vi "UI Main.vi"() -> ()   [LabVIEW 2013]
uses:
  controls/UI Data.ctl
  Globals/Global - All UI Loop Stop.vi
  support/Message Queue/Message Queue.lvlib
  support/User Event - Stop/User Event - Stop.lvlib
panel:
  out "Error Infomation":string caption="错误信息"
  in  "Connect to Controller":bool caption="连接控制器"
  out "Controller Operating Status":u16(ring)=1 caption="控制器运行状态" items=["采集与记录", "安全状态"]
  out "Connected?":bool caption="已连接？"
  in  "Controller Address":string="169.254.4.42" caption="控制器地址"
  in  "Settings Tab":enum32{"采集与记录", "System Monitoring"}(tab) caption="设置选项卡"
  in  "Manually Trigger Data Logging":bool caption="人为触发数据采集"
  out "Live Data":waveform(dbl)[](graph) caption="实时数据"
  in  "Acquire Live Data":bool caption="获取实时数据"
  out "Latest Data Logging File":path=path "最新数据记录文件" caption="最新数据记录文件"
  out "Number of Data Files":u32 caption="数据文件数："
  out "Actual Loop Period (ticks)":u32 caption="实际循环周期（时钟滴答）："
  out "Largest Contiguous Memory (bytes)":dbl(graph) caption="最大连续内存（字节）"
  out "System Time":timestamp caption="系统时间" format="%<%Y/%m/%d %H:%M:%S>T"
  out "Resource Utilization (%)":T1(graph) caption="资源利用率(%)"
  in  "Exit":bool caption="退出"
  # "CompactRIO上的LabVIEW FPGA波形采集与记录"
  # "连接设置"
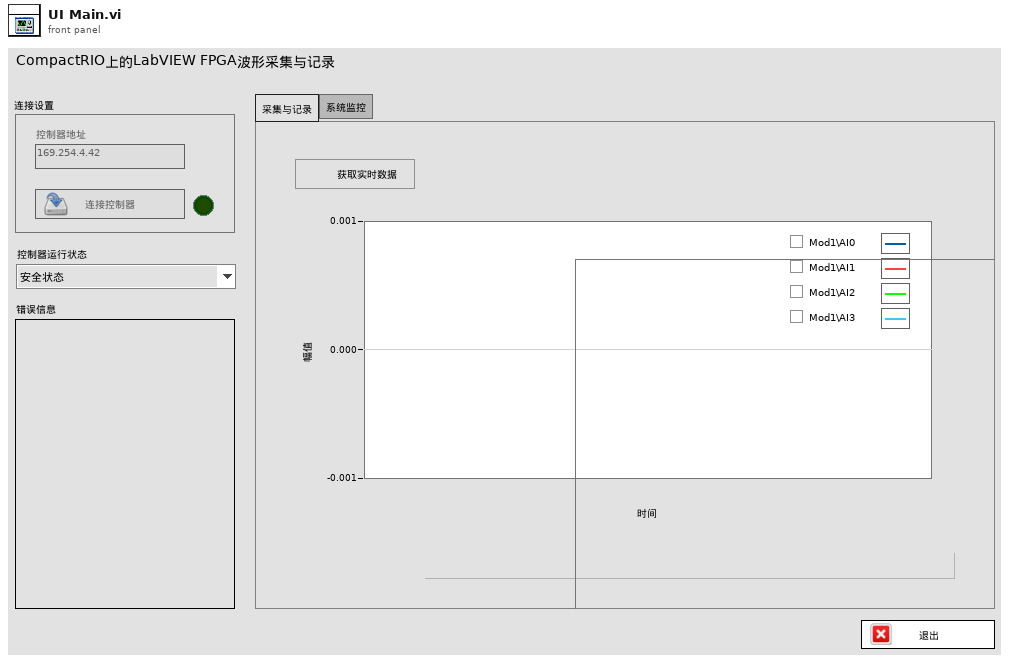
[diagram p1: front panel]
types:
  T1 = cluster{"CPU Usage":dbl, "Buffer Backlog":dbl, "Driver Space":dbl}
  T2 = typedef "UI Data.ctl" = cluster{"Connect to Controller Ref":refnum<vi>, "Connected? Ref":refnum<vi>, "Manually Trigger Data Logging Ref":refnum<vi>, "Acquire Live Data Ref":refnum<vi>, "Stop Live Data Ref":refnum<vi>, "Exit":refnum<vi>, "Controller Address Ref":refnum<vi>, "Error Infomation Ref":refnum<vi>, "Latest Data Logging File Ref":refnum<vi>, "Current Logging State Ref":refnum<vi>, "Actual Loop Period (ticks) Ref":refnum<vi>, "Number of Data Files Ref":refnum<vi>, "System Time Ref":refnum<vi>, "Contiguous Memory Ref":refnum<vi>, "Resource Utilization (%) Ref":refnum<vi>, "Live Data Ref":refnum<vi>, "Setting Tab Ref ":refnum<vi>}
  T3 = typedef "Message Queue.lvlib/All Host Message Queues.ctl" = cluster{"UI":refnum<queue>}
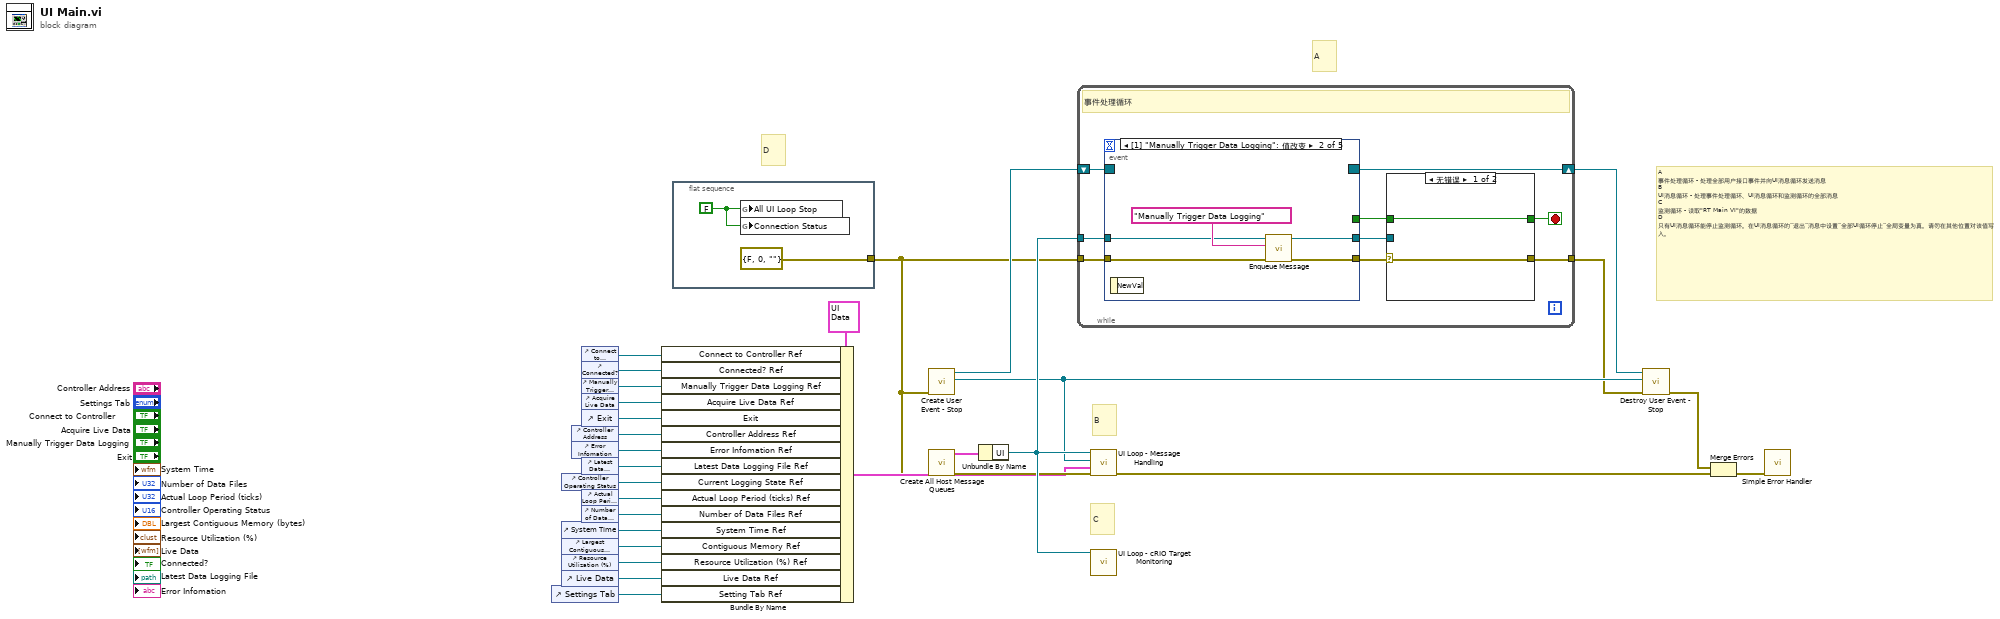
[diagram p0: block diagram]
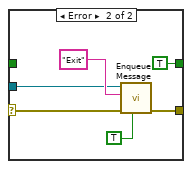
[diagram p2: hidden frame]
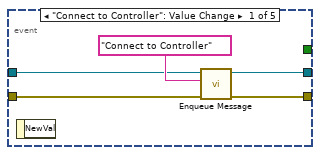
[diagram p3: hidden frame]
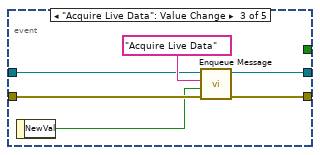
[diagram p4: hidden frame]
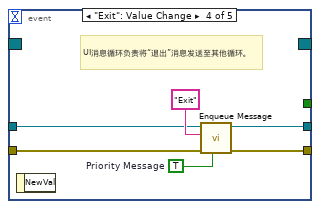
[diagram p5: hidden frame]
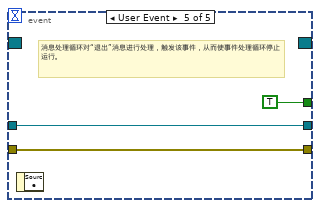
[diagram p6: hidden frame]
diagram:
  # "C"
  # "A"
  # "B"
  # "D"
  # "A\n事件处理循环 - 处理全部用户接口事件并向UI消息循环发送消息\nB\nUI消息循环 - 处理事件处理循环、UI消息循环和监测循环的全部消息\nC\n监测循环 - 读取\"RT Main VI\"的数据\nD\n只有UI消息循环能停止监测循环。在UI消息循环的“退出”消息中设置“全部UI循环停止”全局变量为真。请勿在其他位置对该值写入。"
  n1 = control-ref of="Settings Tab"() -> (w1:refnum<vi>)
  n2 = control-ref of="Controller Operating Status"() -> (w8:refnum<vi>)
  n3 = control-ref of="System Time"() -> (w5:refnum<vi>)
  n4 = control-ref of="Largest Contiguous Memory (bytes)"() -> (w4:refnum<vi>)
  n5 = control-ref of="Resource Utilization (%)"() -> (w3:refnum<vi>)
  n6 = control-ref of="Live Data"() -> (w2:refnum<vi>)
  n7 = control-ref of="Controller Address"() -> (w18:refnum<vi>)
  n8 = control-ref of="Error Infomation"() -> (w9:refnum<vi>)
  n9 = control-ref of="Connect to Controller"() -> (w23:refnum<vi>)
  n10 = control-ref of="Connected?"() -> (w22:refnum<vi>)
  n11 = control-ref of="Manually Trigger Data Logging"() -> (w21:refnum<vi>)
  n12 = control-ref of="Acquire Live Data"() -> (w20:refnum<vi>)
  n13 = control-ref of="Exit"() -> (w19:refnum<vi>)
  n14 = control-ref of="Latest Data Logging File"() -> (w17:refnum<vi>)
  n15 = control-ref of="Actual Loop Period (ticks)"() -> (w7:refnum<vi>)
  n16 = control-ref of="Number of Data Files"() -> (w6:refnum<vi>)
  n17 = Bundle By Name(cluster=T2 {"Connect to Controller Ref"=refnum, "Connected? Ref"=refnum, "Manually Trigger Data Logging Ref"=refnum, "Acquire Live Data Ref"=refnum, "Stop Live Data Ref"=refnum, "Exit"=refnum, "Controller Address Ref"=refnum, "Error Infomation Ref"=refnum, "Latest Data Logging File Ref"=refnum, "Current Logging State Ref"=refnum, "Actual Loop Period (ticks) Ref"=refnum, "Number of Data Files Ref"=refnum, "System Time Ref"=refnum, "Contiguous Memory Ref"=refnum, "Resource Utilization (%) Ref"=refnum, "Live Data Ref"=refnum, "Setting Tab Ref "=refnum} ("Measurement UI Controls"), "Connect to Controller Ref"=w23, "Connected? Ref"=w22, "Manually Trigger Data Logging Ref"=w21, "Acquire Live Data Ref"=w20, "Exit"=w19, "Controller Address Ref"=w18, "Error Infomation Ref"=w9, "Latest Data Logging File Ref"=w17, "Current Logging State Ref"=w8, "Actual Loop Period (ticks) Ref"=w7, "Number of Data Files Ref"=w6, "System Time Ref"=w5, "Contiguous Memory Ref"=w4, "Resource Utilization (%) Ref"=w3, "Live Data Ref"=w2, "Setting Tab Ref"=w1) -> (w12:T2)
  n18 = flat-sequence {
    tunnel: [errorcluster {"status"=FALSE, "code"=0, "source"=""} ("error in (no error)")] -> w11
    frame #0 {
      w30 = FALSE
      n19 = global write "Global - All UI Loop Stop.vi" "All UI Loop Stop"(w30) -> ()
      n20 = global write "Global - All UI Loop Stop.vi" "Connection Status"(w30) -> ()
    }
  }
  n21 = call "Create User Event - Stop.vi"("error in (no error)"=w11) -> ("User Event - Stop"=w15:refnum<user-event>, "Stop Event Registration Refnum"=w29:refnum<event-registration>)  [unwired: 8 in, 1 out]
  n22 = call "Create All Host Message Queues.vi"("error in (no error)"=w11) -> ("error out"=w26:errorcluster, "Message Queues out"=w28:T3)  [unwired: 9 in]
  n23 = Unbundle By Name(w28) -> ("UI"=w27:refnum<queue>)
  n24 = while {
    tunnel: w27 -> [w36]
    shift-right: [w35] -> w13
    shift-left: w29 -> [w37]
    tunnel: w11 -> [w34]
    tunnel: [w32] -> w10
    stop <- w39 stop-if-true
    # "事件处理循环"
    n25 = event shown="[1] \"Manually Trigger Data Logging\": 值改变" {
      selector: w37 -> [_ _ _ _ _]
      dyn-events: [_ _ _ _ _] -> w35
      timeout: _ -> [_ _ _ _ _]
      tunnel: [_ _ _ _ TRUE ("Discard?")] -> w40
      tunnel: w36 -> [w51 w56 w62 w67 w71]
      tunnel: [w53 w58 w64 w70 w72] -> w38
      tunnel: w34 -> [w50 w55 w61 w66 w72]
      tunnel: [w49 w54 w60 w65 w71] -> w33
      event "Connect to Controller": Value Change {
        n26 = event-data() -> ()  [unwired: 1 in, 1 out]
        n27 = call "Enqueue Message.vi"("error in (no error)"=w50, "Message"="Connect to Controller", "Message Queue"=w51) -> ("error out"=w53:errorcluster, "dup Message Queue"=w49:refnum<queue>)  [unwired: 7 in]
      }
      event "Manually Trigger Data Logging": Value Change {
        n28 = event-data() -> ()  [unwired: 1 in, 1 out]
        n29 = call "Enqueue Message.vi"("error in (no error)"=w55, "Message"="Manually Trigger Data Logging", "Message Queue"=w56) -> ("error out"=w58:errorcluster, "dup Message Queue"=w54:refnum<queue>)  [unwired: 7 in]
      }
      event "Acquire Live Data": Value Change {
        n30 = event-data() -> ("NewVal"=w59:bool)  [unwired: 1 in]
        n31 = call "Enqueue Message.vi"("error in (no error)"=w61, "Message Data"=w59, "Message"="Acquire Live Data", "Message Queue"=w62) -> ("error out"=w64:errorcluster, "dup Message Queue"=w60:refnum<queue>)  [unwired: 6 in]
      }
      event "Exit": Value Change {
        w68 = TRUE  # Priority Message
        # "UI消息循环负责将“退出”消息发送至其他循环。"
        n32 = event-data() -> ()  [unwired: 1 in, 1 out]
        n33 = call "Enqueue Message.vi"("Priority Message? (F)"=w68, "error in (no error)"=w66, "Message"="Exit", "Message Queue"=w67) -> ("error out"=w70:errorcluster, "dup Message Queue"=w65:refnum<queue>)  [unwired: 6 in]
      }
      event User Event {
        # "消息处理循环对“退出”消息进行处理，触发该事件，从而使事件处理循环停止运行。"
        n34 = event-data() -> ()  [unwired: 1 in, 1 out]
      }
    }
    n35 = case shown="无错误" w38 {
      selector: w38 -> [w41 w44]
      tunnel: [w42 TRUE ("Discard?")] -> w39
      tunnel: w40 -> [w42 _]
      tunnel: w33 -> [_ w45]
      tunnel: [w41 w43] -> w32
      frame No Error {
        # "无错误"
      }
      frame Error {
        # "出现错误时，发送“退出”消息，使循环停止运行。"
        n36 = call "Enqueue Message.vi"("Priority Message? (F)"=TRUE ("Discard?"), "error in (no error)"=w44, "Message"="Exit", "Message Queue"=w45) -> ("error out"=w43:errorcluster)  [unwired: 6 in, 1 out]
      }
    }
  }
  n37 = call "UI Loop - Message Handling.vi"("error in (no error)"=w26, "UI Control Refs Cluster"=w12, "User Event - Stop"=w15, "UI Message Queue Ref"=w27) -> ("error out"=w25:errorcluster)  [unwired: 7 in]
  n38 = call "UI Loop - cRIO Target Monitoring.vi"("Message Queue Reference"=w27) -> ()  [unwired: 11 in]
  n39 = call "Destroy User Event - Stop.vi"("Stop Event Registeration"=w13, "User Event - Stop"=w15, "error in (no error)"=w10) -> ("error out"=w14:errorcluster)  [unwired: 7 in]
  n40 = Merge Errors(w14, w25) -> (w16:errorcluster)
  n41 = call <vilib>:"Simple Error Handler.vi"("error in (no error)"=w16) -> ()  [unwired: 4 in, 5 out]
